vi "Shoot Balls.vi"(11 "Use Kinect?":bool) -> (3 "Shot All Balls?":bool)   [LabVIEW 2011]
uses:
  Team Code/Robot Global Data.vi
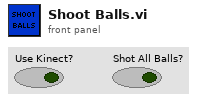
[diagram p1: front panel]
types:
  T1 = cluster{"Left Arm":dbl, "Right Arm":dbl, "Head Right":bool, "Head Left":bool, "Right Leg to Right":bool, "Left Leg to Left":bool, "Right Leg Forward":bool, "Right Leg Back":bool, "Left Leg Forward":bool, "Left Leg Back":bool, "Enable":bool, "Distance":dbl, "Enable Override?":bool, "FIRE!!!!":bool}
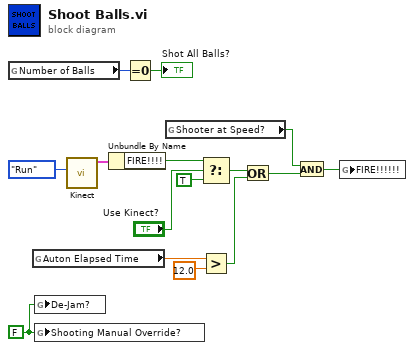
[diagram p0: block diagram]
diagram:
  w3 = FALSE ("De-Jam?")
  n1 = global read "Robot Global Data.vi" "Number of Balls"() -> (w1:i32)
  n2 = global read "Robot Global Data.vi" "Auton Elapsed Time"() -> (w6:dbl)
  n3 = global write "Robot Global Data.vi" "De-Jam?"(w3) -> ()
  n4 = global write "Robot Global Data.vi" "Shooting Manual Override?"(w3) -> ()
  n5 = call "Kinect.vi"("Mode"=enum16{"Init", "Run", "End"}."Run") -> ("Kinect"=w14:T1)  [unwired: 10 in]
  n6 = Unbundle By Name(w14) -> ("FIRE!!!!"=w4:bool)
  n7 = Equal To 0?(x=w1) -> (x = 0?=→"Shot All Balls?":bool)
  n8 = global read "Robot Global Data.vi" "Shooter at Speed?"() -> (w5:bool)
  n9 = Select(t=w4, s="Use Kinect?", f=TRUE) -> (s? t:f=w9:bool)
  n10 = Greater?(x=w6, y=12.0 ("x")) -> (0:w10:bool)
  n11 = Or(x=w9, y=w10) -> (x .or. y?=w8:bool)
  n12 = And(x=w5, y=w8) -> (x .and. y?=w2:bool)
  n13 = global write "Robot Global Data.vi" "FIRE!!!!!!"(w2) -> ()
